vi "PH_Timing.ProcEvents.vi"(0 "i ref in":refnum<vi>, 5 "error in":errorcluster) -> (14 "i ref out":refnum<vi>, 19 "error out":errorcluster)   [LabVIEW 2014, in "PH_Timing.lvlib"]
doc: "This method is used to define the events the object will listen to. Add your own events here."
uses:
  PH_Timing.lvlib
  CS_Core/BaseProcess/BaseProcess.event definition.ctl
  CS_Core/CAEObj/CAEObj.event definition.ctl
  CS_Core/BaseProcess/BaseProcess.descriptor string definition.ctl
  PH_Basics/PH_PowerUnit_BaseClass/PH_PowerUnit_BaseClass.PP PU Tags.ctl
  CS_Core/BaseProcess/BaseProcess.lvlib
  CS_Core/CAEObj/CAEObj.lvlib
  PH_Basics/PH_Common/PH_Common.lvlib
  PH_Basics/PH_PowerUnit_BaseClass/PH_PowerUnit_BaseClass.lvlib
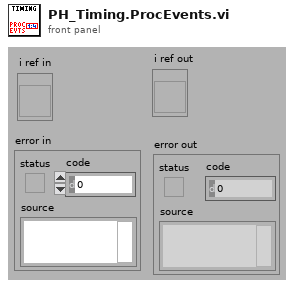
[diagram p1: front panel]
types:
  T1 = typedef "BaseProcess.lvlib/BaseProcess.event definition.ctl" = cluster{"CAEEvtDef":T2, "Data Descriptor":T3}
  T2 = typedef "CAEObj.lvlib/CAEObj.event definition.ctl" = cluster{"URL":string, "enable":bool, "ignoreResID":bool}
  T3 = typedef "BaseProcess.lvlib/BaseProcess.descriptor string definition.ctl" = string
  T4 = typedef "PH_PowerUnit_BaseClass.lvlib/PH_PowerUnit_BaseClass.PP PU Tags.ctl" = enum16{"Waiting-Time", "PU-in-Use"}
  T5 = typedef "PH_Timing.lvlib/PH_Timing.i attribute.ctl" = cluster{"Sequencer":cluster{"linked?":bool, "Proc State":string, "Ref State":refnum<vi>}, "Gate Generator":cluster{"GD":cluster{"Device Status":T6, "linked?":bool}, "Settings":T7, "GUI Ref":refnum<vi>}, "Interlock Bypass":cluster{"Instancename":string, "Switch linked?":bool, "Device Status":T6, "Ref Status":refnum<vi>}, "Roughtuner":cluster{"Settings":T8, "GUI Ref":refnum<vi>, "GD":cluster{"Device Status":T6, "linked?":bool}}, "0,5Hz Gater":cluster{"Settings":T9, "GUI Ref":refnum<vi>, "GD":cluster{"Device Status":T6, "linked?":bool}}, "Slow Trigger":cluster{"Settings":T10, "GUI Ref":refnum<vi>, "Service ID Delay":i32, "Service ID Ext Trig":i32, "Wanted Settings":T10}, "Timing Mode":cluster{"Mode":T11, "GUI Ref":refnum<vi>, "Service ID T2":i32, "Service ID Mode":i32, "Wanted Mode":T11}, "ns Generator":cluster{"Settings":T12, "ns Generator Settings":refnum<vi>, "GD":cluster{"Device Status":T6, "linked?":bool}}, "Phase FEs":cluster{"Settings":T15, "GUI Ref":refnum<vi>, "Service ID Phase":i32, "Wanted Settings":T15}, "GD GUI Refs":refnum<vi>[], "Heads":T16[], "GUI Ref Delete":refnum<vi>}
  T6 = typedef "PH_StatusHandler.lvlib/PH_StatusHandler.Status.ctl" = i16
  T7 = typedef "PH_Timing.lvlib/PH_Timing.GateGen.ctl" = cluster{"Instance":string, "Channel Gate":i32, "Channel T2":i32, "Width Gate":dbl, "Width T2":dbl, "Delay Gate":dbl, "Delay T2":dbl, "Gate activ":bool, "T2 activ":bool, "System Mode":enum16{"Normal", "Single", "Burst", "Duty Cycle"}}
  T8 = typedef "PH_Timing.lvlib/PH_Timing.Roughtuner.ctl" = cluster{"Instance":string, "Phase PHELIX / UNILAC":cluster{"Channel":u16, "relative to":u16, "Delay [ms]":dbl}, "Pulse Length":cluster{"Channel":u16, "relative to":u16, "Delay [ms]":dbl}, "Trigger":cluster{"externally?":bool, "Rate [Hz]":dbl}}
  T9 = typedef "PH_Timing.lvlib/PH_Timing.0.5HzGater.ctl" = cluster{"Instance":string, "Channel ns FE Delay":i32, "Channel 0.5Hz":i32, "Width ns FE Delay":dbl, "Width 0.5Hz":dbl, "Delay ns FE Delay":dbl, "Delay 0.5Hz":dbl, "ns FE Delay active":bool, "0.5Hz activ":bool, "ns FE Delay inverted":bool, "0.5Hz inverted":bool}
  T10 = typedef "PH_Timing.lvlib/PH_Timing.Slow Trigger Settings.ctl" = cluster{"Delay":dbl, "externally triggered?":bool}
  T11 = typedef "PH_Timing.lvlib/PH_Timing.Timing Mode.ctl" = cluster{"T2":i16, "Modeselector":enum32{"10 Hz", "0.5 Hz", "Shot"}}
  T12 = typedef "PH_Timing.lvlib/PH_Timing.ns Generator.ctl" = cluster{"Instance":string, "Phase fs / ns FE":cluster{"Channel":T13, "Settings":T14}}
  T13 = typedef "Stanford Research DG645 - Driver.lvlib/Channel.ctl" = i32
  T14 = typedef "PH_SRDG645.lvlib/PH_SRDG645.Channel Settings.ctl" = cluster{"Delay [s]":dbl, "relative to":i32}
  T15 = typedef "PH_Timing.lvlib/PH_Timing.Phase FEs.ctl" = cluster{"Phase":dbl}
  T16 = typedef "PH_Timing.lvlib/PH_Timing.PU Data.ctl" = cluster{"linked?":bool, "Data":T17, "GD":cluster{"Device Status":T6, "linked?":bool}, "GUI Ref":refnum<vi>, "PU":T18}
  T17 = typedef "PH_Timing.lvlib/PH_Timing.PU Info.ctl" = cluster{"Act CH?":bool, "GD":string, "CH":i32, "Delay":dbl, "active":bool, "in Use?":bool}
  T18 = typedef "PH_PP_Common.lvlib/PH_PP_Common.PUs.ctl" = enum16{"no Info", "PA-19mm-1", "PA-19mm-2", "PA-45mm-PILC", "PA-45mm-MAIN", "MA-PU-1", "MA-PU-2", "MA-PU-3", "MA-PU-4", "MA-PU-5", "MA-PU-6", "MA-FR", "MA-PILC", "PA-45mm-DP"}
  T19 = typedef "PH_Common.lvlib/PH_DIM.Event Declarer.ctl" = cluster{"Service Name":string, "Selector":string}
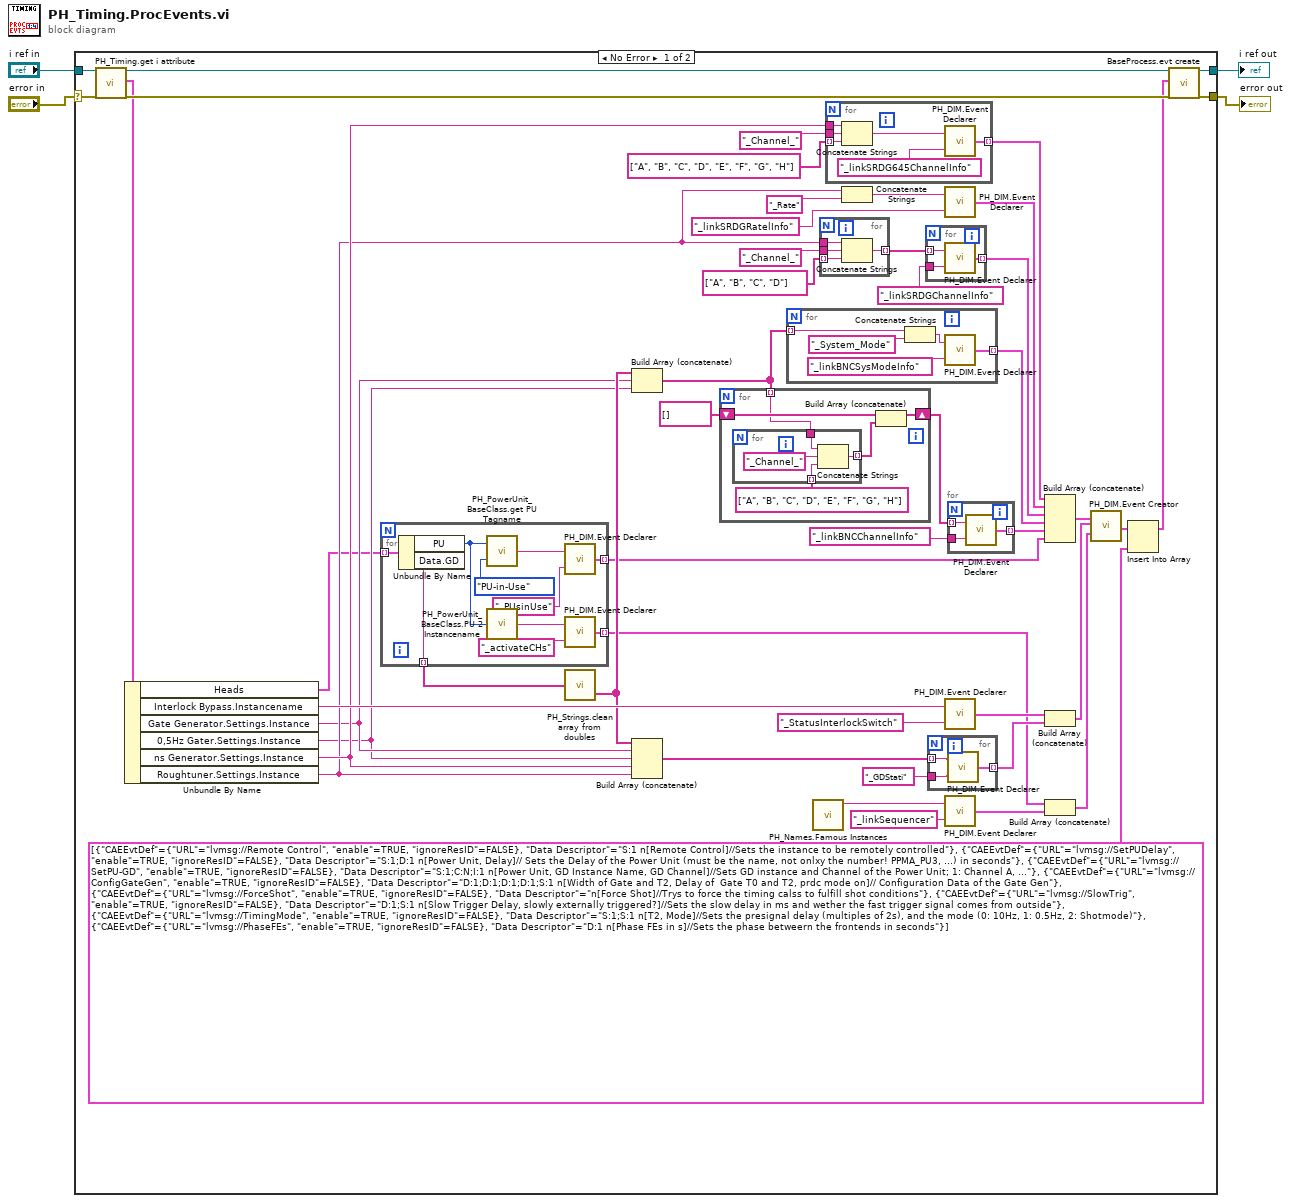
[diagram p0: block diagram]
diagram:
  n1 = case shown="No Error" "error in" {
    selector: "error in" -> [w51 w97]
    tunnel: "i ref in" -> [w49 w98]
    tunnel: [w53 w98] -> w3
    tunnel: [w52 w97] -> w2
    frame No Error {
      n2 = call "PH_Timing.get i attribute.vi"("i ref in"=w49, "error in (no error)"=w51) -> ("i ref out"=w48:refnum<vi>, "i attribute"=w47:T5, "error out"=w50:errorcluster)  [unwired: 15 in]
      n3 = Unbundle By Name(w47) -> ("Heads"=w8:T16[], "Interlock Bypass.Instancename"=w25:string, "Gate Generator.Settings.Instance"=w10:string, "0,5Hz Gater.Settings.Instance"=w9:string, "ns Generator.Settings.Instance"=w15:string, "Roughtuner.Settings.Instance"=w14:string)
      n4 = for {
        tunnel: w8 -> [w93] mode=indexing
        tunnel: [w91] -> w6 mode=indexing
        tunnel: [w87] -> w5 mode=indexing
        tunnel: [w86] -> w12 mode=indexing
        n5 = Unbundle By Name(w93) -> ("PU"=w85:T18, "Data.GD"=w86:string)
        n6 = call "PH_PowerUnit_BaseClass.get PU Tagname.vi"("PU Tag"=PH_PowerUnit_BaseClass.PP_PU_Tags."PU-in-Use", "PU"=w85) -> ("PU Tagname"=w88:string)
        n7 = call "PH_PowerUnit_BaseClass.PU 2 Instancename.vi"("PU"=w85) -> ("Instance Name"=w84:string)
        n8 = call "PH_DIM.Event Declarer.vi"("Selector"="_PUsinUse", "Service Name"=w88) -> ("declared DIM Event"=w87:T19)
        n9 = call "PH_DIM.Event Declarer.vi"("Selector"="_activateCHs" ("URL"), "Service Name"=w84) -> ("declared DIM Event"=w91:T19)
      }
      n10 = call "PH_Strings.clean array from doubles.vi"("Array Input"=w12) -> ("Cleaned Array Output"=w11:string[])  [unwired: 1 out]
      n11 = Build Array (concatenate)(w11, w10, w9) -> (w30:string[])
      n12 = Build Array (concatenate)(w11, w10, w9, w15, w14) -> (w16:string[])
      n13 = for {
        shift-right: [w78] -> w41
        shift-left: string[] [] -> [w77]
        tunnel: w30 -> [w76] mode=indexing
        n14 = for {
          tunnel: string[] ["A", "B", "C", "D", "E", "F", "G", "H"] -> [w82] mode=indexing
          tunnel: [w81] -> w75 mode=indexing
          tunnel: w76 -> [w80]
          n15 = Concatenate Strings(w80, "_Channel_" ("string"), w82) -> (w81:string)
        }
        n16 = Build Array (concatenate)(w77, w75) -> (w78:string[])
      }
      n17 = for {
        tunnel: w30 -> [w63] mode=indexing
        tunnel: [w61] -> w29 mode=indexing
        n18 = Concatenate Strings(w63, "_System_Mode" ("Service Name")) -> (w62:string)
        n19 = call "PH_DIM.Event Declarer.vi"("Selector"="_linkBNCSysModeInfo" ("URL"), "Service Name"=w62) -> ("declared DIM Event"=w61:T19)
      }
      n20 = call "PH_Names.Famous Instances.vi"() -> ("Sequencer"=w7:string)  [unwired: 7 in, 3 out]
      n21 = for {
        tunnel: string[] ["A", "B", "C", "D"] -> [w71] mode=indexing
        tunnel: "_Channel_" ("string") -> [w70]
        tunnel: [w69] -> w35 mode=indexing
        tunnel: w14 -> [w68]
        n22 = Concatenate Strings(w68, w70, w71) -> (w69:string)
      }
      n23 = for {
        tunnel: w15 -> [w59]
        tunnel: "_Channel_" ("string") -> [w58]
        tunnel: [w56] -> w20 mode=indexing
        tunnel: string[] ["A", "B", "C", "D", "E", "F", "G", "H"] -> [w55] mode=indexing
        n24 = Concatenate Strings(w59, w58, w55) -> (w57:string)
        n25 = call "PH_DIM.Event Declarer.vi"("Selector"="_linkSRDG645ChannelInfo", "Service Name"=w57) -> ("declared DIM Event"=w56:T19)
      }
      n26 = Concatenate Strings(w14, "_Rate" ("string")) -> (w28:string)
      n27 = for {
        tunnel: [w66] -> w32 mode=indexing
        tunnel: w35 -> [w67] mode=indexing
        tunnel: "_linkSRDGChannelInfo" -> [w65]
        n28 = call "PH_DIM.Event Declarer.vi"("Selector"=w65, "Service Name"=w67) -> ("declared DIM Event"=w66:T19)
      }
      n29 = for {
        tunnel: [w96] -> w23 mode=indexing
        tunnel: w16 -> [w95] mode=indexing
        tunnel: "_GDStati" ("URL") -> [w94]
        n30 = call "PH_DIM.Event Declarer.vi"("Selector"=w94, "Service Name"=w95) -> ("declared DIM Event"=w96:T19)
      }
      n31 = call "PH_DIM.Event Declarer.vi"("Selector"="_linkSRDGRatelInfo", "Service Name"=w28) -> ("declared DIM Event"=w26:T19)
      n32 = call "PH_DIM.Event Declarer.vi"("Selector"="_StatusInterlockSwitch" ("URL"), "Service Name"=w25) -> ("declared DIM Event"=w22:T19)
      n33 = call "PH_DIM.Event Declarer.vi"("Selector"="_linkSequencer" ("URL"), "Service Name"=w7) -> ("declared DIM Event"=w43:T19)
      n34 = for {
        tunnel: [w72] -> w31 mode=indexing
        tunnel: w41 -> [w74] mode=indexing
        tunnel: "_linkBNCChannelInfo" ("URL") -> [w73]
        n35 = call "PH_DIM.Event Declarer.vi"("Selector"=w73, "Service Name"=w74) -> ("declared DIM Event"=w72:T19)
      }
      n36 = Build Array (concatenate)(w20, w26, w32, w29, w31, w5) -> (w34:T19[])
      n37 = Build Array (concatenate)(w22, w23) -> (w42:T19[])
      n38 = Build Array (concatenate)(w6, w43) -> (w17:T19[])
      n39 = call "PH_DIM.Event Creator.vi"("Trendmessage Services"=w34, "Status Services"=w42, "SM State Services"=w17) -> ("DIM Service Events"=w44:T1[])  [unwired: 16 in]
      n40 = Insert Into Array(array=w44, new element=T1[] [{"CAEEvtDef"={"URL"="lvmsg://Remote Control", "enable"=TRUE, "ignoreResID"=FALSE}, "Data Descriptor"="S:1 n[Remote Control]//Sets the instance to be remotely controlled"}, {"CAEEvtDef"={"URL"="lvmsg://SetPUDelay", "enable"=TRUE, "ignoreResID"=FALSE}, "Data Descriptor"="S:1;D:1 n[Power Unit, Delay]// Sets the Delay of the Power Unit (must be the name, not onlxy the number! PPMA_PU3, ...) in seconds"}, {"CAEEvtDef"={"URL"="lvmsg://SetPU-GD", "enable"=TRUE, "ignoreResID"=FALSE}, "Data Descriptor"="S:1;C:N;I:1 n[Power Unit, GD Instance Name, GD Channel]//Sets GD instance and Channel of the Power Unit; 1: Channel A, ..."}, {"CAEEvtDef"={"URL"="lvmsg://ConfigGateGen", "enable"=TRUE, "ignoreResID"=FALSE}, "Data Descriptor"="D:1;D:1;D:1;D:1;S:1 n[Width of Gate and T2, Delay of  Gate T0 and T2, prdc mode on]// Configuration Data of the Gate Gen"}, {"CAEEvtDef"={"URL"="lvmsg://ForceShot", "enable"=TRUE, "ignoreResID"=FALSE}, "Data Descriptor"="n[Force Shot]//Trys to force the timing calss to fulfill shot conditions"}, {"CAEEvtDef"={"URL"="lvmsg://SlowTrig", "enable"=TRUE, "ignoreResID"=FALSE}, "Data Descriptor"="D:1;S:1 n[Slow Trigger Delay, slowly externally triggered?]//Sets the slow delay in ms and wether the fast trigger signal comes from outside"}, {"CAEEvtDef"={"URL"="lvmsg://TimingMode", "enable"=TRUE, "ignoreResID"=FALSE}, "Data Descriptor"="S:1;S:1 n[T2, Mode]//Sets the presignal delay (multiples of 2s), and the mode (0: 10Hz, 1: 0.5Hz, 2: Shotmode)"}, {"CAEEvtDef"={"URL"="lvmsg://PhaseFEs", "enable"=TRUE, "ignoreResID"=FALSE}, "Data Descriptor"="D:1 n[Phase FEs in s]//Sets the phase betweern the frontends in seconds"}] ("new events")) -> (w46:T1[])  [unwired: 1 in]
      n41 = call "BaseProcess.evt create.vi"("i ref in"=w48, "newEvents"=w46, "error in (no error)"=w50) -> ("i ref out"=w53:refnum<vi>, "error out"=w52:errorcluster)  [unwired: 13 in, 2 out]
    }
    frame Error {
    }
  }
  "i ref out" <- w3
  "error out" <- w2
